vi "Translator.File.GetDefaultStrings (Array).vi"(5 "refnum in":T1, 7 "group":string, 8 "error in":errorcluster, 9 "labels":string[](array[string]), 10 "default values":string[](array[string])) -> (0 "error out":errorcluster, 2 "values out":string[](array[string]))   [LabVIEW 2019, in "Tools.lvlib"]
uses:
  Tools.lvlib
  <vilib>/Utility/config.llb/Config Data RefNum.ctl
  <vilib>/Utility/config.llb/Read Key (String).vi
  <vilib>/Utility/config.llb/NI_LVConfig.lvlib
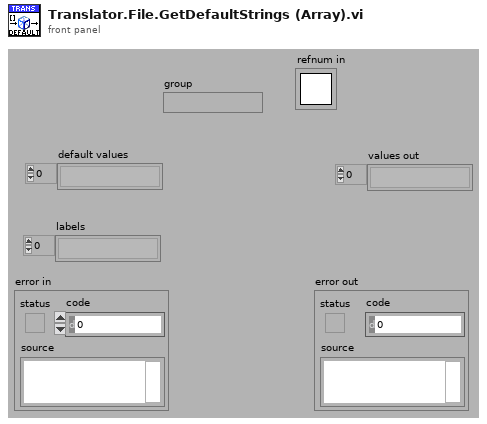
[diagram p1: front panel]
types:
  T1 = typedef "NI_LVConfig.lvlib/Config Data RefNum.ctl" = refnum<k1>
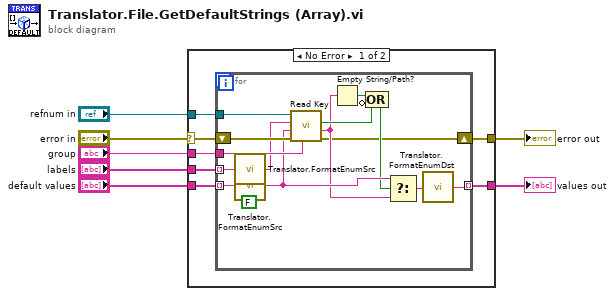
[diagram p0: block diagram]
diagram:
  n1 = case shown="No Error" "error in" {
    selector: "error in" -> [w10 w31]
    tunnel: "refnum in" -> [w9 _]
    tunnel: [w14 w31] -> w7
    tunnel: [w13 w30] -> w6
    tunnel: "group" -> [w12 _]
    tunnel: "labels" -> [w8 _]
    tunnel: "default values" -> [w11 w30]
    frame No Error {
      n2 = for {
        tunnel: w12 -> [w27]
        tunnel: w8 -> [w26] mode=indexing
        shift-right: [w15] -> w14
        shift-left: w10 -> [w29]
        tunnel: [w17] -> w13 mode=indexing
        tunnel: w11 -> [w25] mode=indexing
        tunnel: w9 -> [w28]
        n3 = call "Translator.FormatEnumSrc.vi"("text in"=w26) -> ("text out"=w18:string)  [unwired: 1 in]
        n4 = call "Translator.FormatEnumSrc.vi"("text in"=w25, "quotas?(T)"=FALSE) -> ("text out"=w24:string)
        n5 = call-poly <vilib>:"Read Key.vi"("section"=w27, "error in (no error)"=w29, "default value"=w24, "key"=w18, "refnum"=w28) -> ("error out"=w15:errorcluster, "value"=w20:string, "found?"=w21:bool)  [unwired: 3 in, 1 out]
        n6 = Empty String/Path?(string/path=w20) -> (empty?=w23:bool)
        n7 = Compound Arithmetic op=OR(w23, invert w21) -> (w22:bool)
        n8 = Select(t=w24, s=w22, f=w20) -> (s? t:f=w16:string)
        n9 = call "Translator.FormatEnumDst.vi"("text in"=w16) -> ("text out"=w17:string)
      }
    }
    frame Error {
    }
  }
  "error out" <- w7
  "values out" <- w6
